vi "shorttolongtime.vi"(0 "object in":refnum<class "interface.lvclass">, 1 "data":string[][](table), 2 "table输入":string(combo), 5 "error in (no error)":errorcluster) -> (14 "object out":refnum<class "interface.lvclass">, 15 "输出数组":string[][](array[string]), 19 "error out":errorcluster)   [LabVIEW 2016, in "interface.lvclass"]
uses:
  interface.lvclass
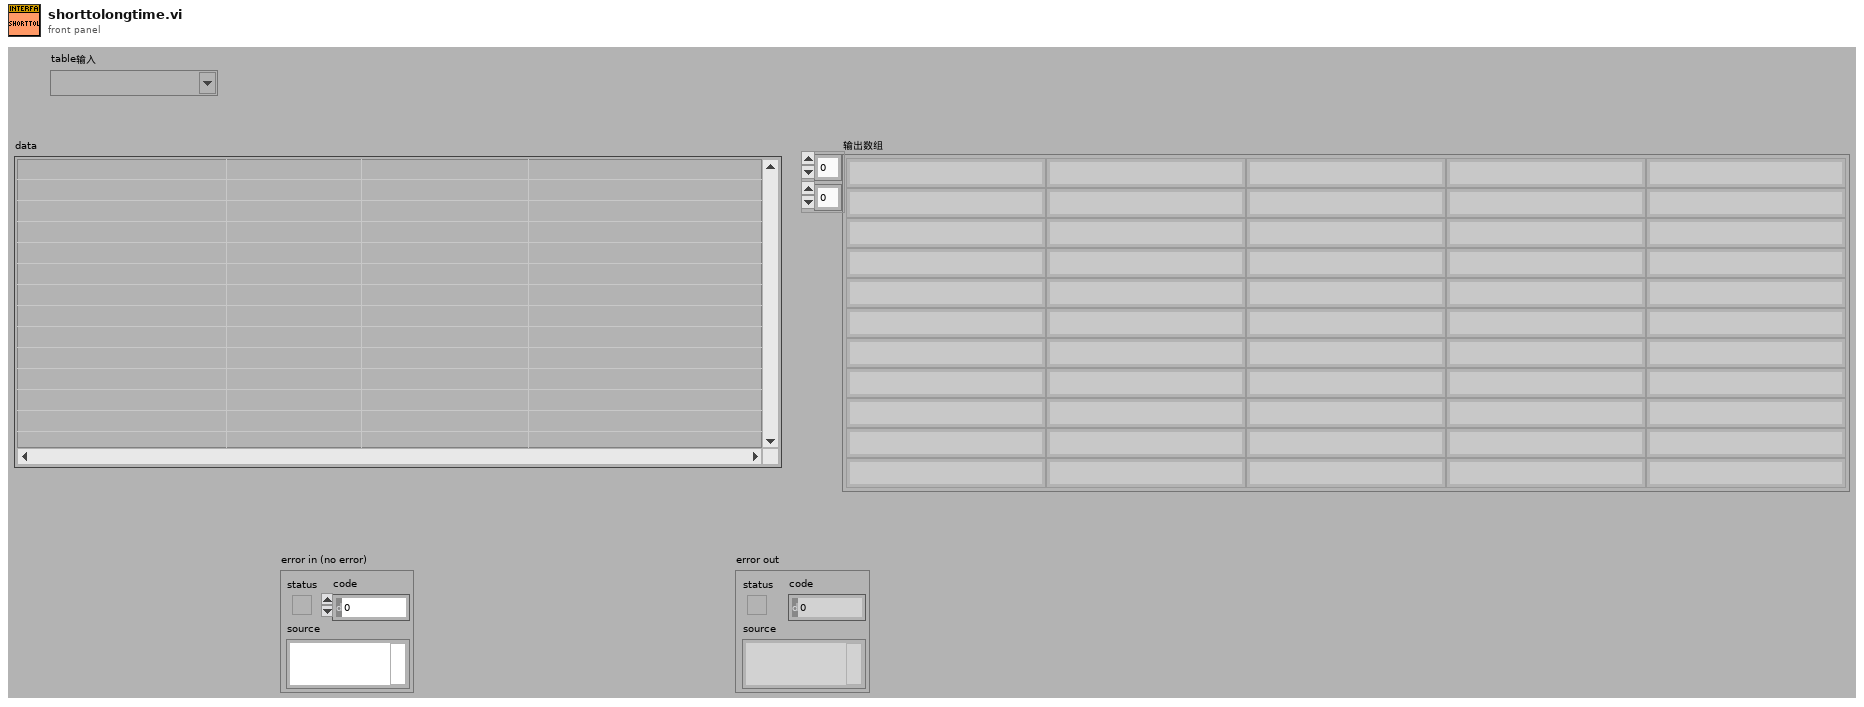
[diagram p1: front panel]
types:
  T1 = typedef "LVDateTimeRec.ctl" = cluster{"秒数的小数部分":dbl, "秒":i32, "分":i32, "时":i32, "日":i32, "月":i32, "年":i32, "天数（周）":i32, "天数（年）":i32, "DST":i32}
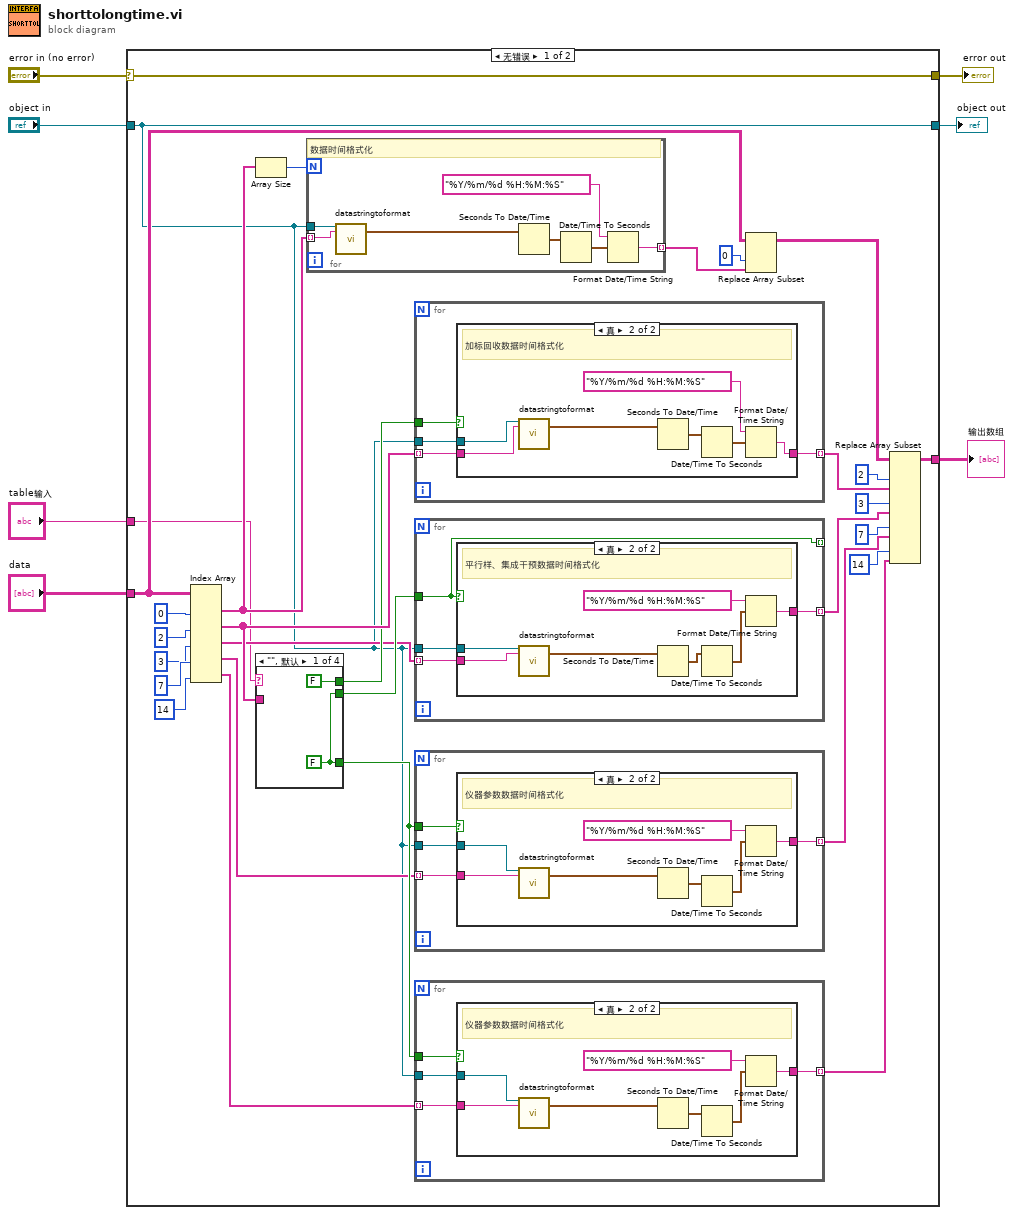
[diagram p0: block diagram]
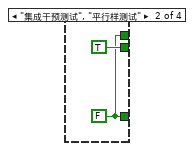
[diagram p6: hidden frame]
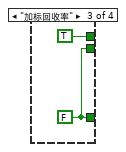
[diagram p7: hidden frame]
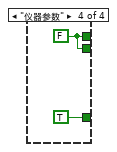
[diagram p8: hidden frame]
diagram:
  n1 = case shown="无错误" "error in (no error)" {
    selector: "error in (no error)" -> [w37 w102]
    tunnel: [w37 w102] -> w6
    tunnel: [w8 w101] -> w4
    tunnel: "object in" -> [w8 w101]
    tunnel: "data" -> [w11 _]
    tunnel: "table输入" -> [w10 _]
    tunnel: [w9 _] -> w1
    frame No Error {
      n2 = Index Array(array=w11, index (col) #1=0 ("禁用的索引 (列)"), index (col) #2=2 ("索引 (列)"), index (col) #3=3 ("索引 (列)"), index (col) #4=7 ("索引 (列)"), index (col) #5=14 ("索引 (列)")) -> (element #1=w30:string[], element #2=w28:string[], element #3=w18:string[], element #4=w23:string[], element #5=w24:string[])  [unwired: 5 in]
      n3 = Array Size(array=w30) -> (size(s)=w29:i32)
      n4 = case shown="\"\", 默认" w10 {
        tunnel: [FALSE w95 TRUE w99] -> w27
        tunnel: w28 -> [_ _ _ _]
        tunnel: [w93 w95 w97 TRUE] -> w25
        tunnel: [w93 TRUE w97 w99] -> w19
        frame "", Default {
          w93 = FALSE
        }
        frame "集成干预测试", "平行样测试" {
          w95 = FALSE
        }
        frame "加标回收率" {
          w97 = FALSE
        }
        frame "仪器参数" {
          w99 = FALSE
        }
      }
      n5 = for {
        N: w29 -> [_]
        tunnel: [w89] -> w33 mode=indexing
        tunnel: w30 -> [w88] mode=indexing
        tunnel: w8 -> [w86]
        # "数据时间格式化"
        n6 = call-dynamic "datastringtoformat.vi"("object in"=w86, "data[0]"=w88) -> ("time stamp"=w87:timestamp)  [unwired: 15 in, 2 out]
        n7 = Seconds To Date/Time(time stamp (now)=w87) -> (date time rec=w92:T1)  [unwired: 1 in]
        n8 = Date/Time To Seconds(2:w92) -> (0:w91:timestamp)  [unwired: 1 in]
        n9 = Format Date/Time String(time format string (%c)="%Y/%m/%d %H:%M:%S" ("时间格式字符串(%c)"), seconds (now)=w91) -> (date/time string=w89:string)  [unwired: 1 in]
      }
      n10 = for {
        tunnel: w28 -> [w53] mode=indexing
        tunnel: w27 -> [w52]
        tunnel: [w51] -> w26 mode=indexing
        tunnel: w8 -> [w50]
        n11 = case shown="真" w52 {
          tunnel: [w54 w58] -> w51
          tunnel: w53 -> [w54 w57]
          tunnel: w50 -> [_ w55]
          frame False {
          }
          frame True {
            # "加标回收数据时间格式化"
            n12 = call-dynamic "datastringtoformat.vi"("object in"=w55, "data[0]"=w57) -> ("time stamp"=w56:timestamp)  [unwired: 15 in, 2 out]
            n13 = Seconds To Date/Time(time stamp (now)=w56) -> (date time rec=w59:T1)  [unwired: 1 in]
            n14 = Date/Time To Seconds(2:w59) -> (0:w60:timestamp)  [unwired: 1 in]
            n15 = Format Date/Time String(time format string (%c)="%Y/%m/%d %H:%M:%S" ("时间格式字符串(%c)"), seconds (now)=w60) -> (date/time string=w58:string)  [unwired: 1 in]
          }
        }
      }
      n16 = for {
        tunnel: w18 -> [w41] mode=indexing
        tunnel: [w39] -> _ mode=indexing
        tunnel: [w40] -> w14 mode=indexing
        tunnel: w19 -> [w39]
        tunnel: w8 -> [w38]
        n17 = case shown="真" w39 {
          tunnel: [w42 w46] -> w40
          tunnel: w41 -> [w42 w45]
          tunnel: w38 -> [_ w43]
          frame False {
          }
          frame True {
            # "平行样、集成干预数据时间格式化"
            n18 = call-dynamic "datastringtoformat.vi"("object in"=w43, "data[0]"=w45) -> ("time stamp"=w44:timestamp)  [unwired: 15 in, 2 out]
            n19 = Seconds To Date/Time(time stamp (now)=w44) -> (date time rec=w47:T1)  [unwired: 1 in]
            n20 = Date/Time To Seconds(2:w47) -> (0:w48:timestamp)  [unwired: 1 in]
            n21 = Format Date/Time String(time format string (%c)="%Y/%m/%d %H:%M:%S" ("时间格式字符串(%c)"), seconds (now)=w48) -> (date/time string=w46:string)  [unwired: 1 in]
          }
        }
      }
      n22 = for {
        tunnel: w23 -> [w65] mode=indexing
        tunnel: [w64] -> w12 mode=indexing
        tunnel: w25 -> [w63]
        tunnel: w8 -> [w62]
        n23 = case shown="真" w63 {
          tunnel: [w66 w70] -> w64
          tunnel: w65 -> [w66 w69]
          tunnel: w62 -> [_ w67]
          frame False {
          }
          frame True {
            # "仪器参数数据时间格式化"
            n24 = call-dynamic "datastringtoformat.vi"("object in"=w67, "data[0]"=w69) -> ("time stamp"=w68:timestamp)  [unwired: 15 in, 2 out]
            n25 = Seconds To Date/Time(time stamp (now)=w68) -> (date time rec=w71:T1)  [unwired: 1 in]
            n26 = Date/Time To Seconds(2:w71) -> (0:w72:timestamp)  [unwired: 1 in]
            n27 = Format Date/Time String(time format string (%c)="%Y/%m/%d %H:%M:%S" ("时间格式字符串(%c)"), seconds (now)=w72) -> (date/time string=w70:string)  [unwired: 1 in]
          }
        }
      }
      n28 = for {
        tunnel: w24 -> [w77] mode=indexing
        tunnel: w25 -> [w76]
        tunnel: [w75] -> w13 mode=indexing
        tunnel: w8 -> [w74]
        n29 = case shown="真" w76 {
          tunnel: [w78 w82] -> w75
          tunnel: w77 -> [w78 w81]
          tunnel: w74 -> [_ w79]
          frame False {
          }
          frame True {
            # "仪器参数数据时间格式化"
            n30 = call-dynamic "datastringtoformat.vi"("object in"=w79, "data[0]"=w81) -> ("time stamp"=w80:timestamp)  [unwired: 15 in, 2 out]
            n31 = Seconds To Date/Time(time stamp (now)=w80) -> (date time rec=w83:T1)  [unwired: 1 in]
            n32 = Date/Time To Seconds(2:w83) -> (0:w84:timestamp)  [unwired: 1 in]
            n33 = Format Date/Time String(time format string (%c)="%Y/%m/%d %H:%M:%S" ("时间格式字符串(%c)"), seconds (now)=w84) -> (date/time string=w82:string)  [unwired: 1 in]
          }
        }
      }
      n34 = Replace Array Subset(array=w11, new element=w33, index (col)=0 ("禁用的索引 (列)")) -> (w31:string[][])  [unwired: 1 in]
      n35 = Replace Array Subset(array=w31, new element #1=w26, index (col) #1=2 ("索引 (列)"), new element #2=w14, index (col) #2=3 ("索引 (列)"), new element #3=w12, index (col) #3=7 ("索引 (列)"), new element #4=w13, index (col) #4=14 ("索引 (列)")) -> (w9:string[][])  [unwired: 4 in]
    }
    frame Error {
    }
  }
  "error out" <- w6
  "object out" <- w4
  "输出数组" <- w1
